vi "LSMcontroller_v59_PIzstage.vi"() -> ()   [LabVIEW 2015] (continued)
                            n1347 = call "reset AO_DO_v3.vi"() -> ()  [unwired: 12 in]
                            n1348 = property on="Start" class="Bool (strict)"("Val(Sgnl)"=w3765) -> ()  [unwired: 2 in, 2 out]
                            n1349 = property on="Start" class="Bool (strict)"("Visible"=TRUE, "DisabledEnum"=T7."Enabled" ("Disabled")) -> ()  [unwired: 2 in, 2 out]
                            n1350 = property on="Stop" class="Bool (strict)"("Val(Sgnl)"=w3765) -> ()  [unwired: 2 in, 2 out]
                            n1351 = property on="Stop" class="Bool (strict)"("Visible"=FALSE, "DisabledEnum"=T7."Disabled" ("Disabled")) -> ()  [unwired: 2 in, 2 out]
                          }
                        }
                      }
                      frame "Line" {
                      }
                      frame "Resonant Ellipse", "freeform contour" {
                        n1352 = stacked-sequence {
                          seq-local: [w3789 _ _ _ _ _ _ _ _ _ _] -> [_ _ w4634 _ _ w4647 w4714 _ _ w5074 _]
                          seq-local: [w3788 _ _ _ _ _ _ _ _ _ _] -> [_ _ _ _ _ _ _ _ w4761 _ _]
                          seq-local: [w3787 _ _ _ _ _ _ _ _ _ _] -> [_ _ _ _ _ _ _ _ w4760 _ _]
                          seq-local: [w3786 _ _ _ _ _ _ _ _ _ _] -> [_ _ _ _ _ _ _ _ w4763 _ _]
                          seq-local: [w3785 _ _ _ _ _ _ _ _ _ _] -> [_ _ _ _ _ _ _ _ w4759 _ _]
                          seq-local: [w3784 _ _ _ _ _ _ _ _ _ _] -> [_ _ _ _ _ _ _ _ w4758 _ _]
                          seq-local: [w3783 _ _ _ _ _ _ _ _ _ _] -> [_ _ _ _ _ _ _ _ w4762 _ _]
                          seq-local: [w3782 _ _ _ _ _ _ _ _ _ _] -> [_ _ _ _ _ _ _ _ w4757 _ _]
                          seq-local: [w3781 _ _ _ _ _ _ _ _ _ _] -> [_ _ _ _ _ _ _ _ w4756 _ _]
                          seq-local: [w3780 _ _ _ _ _ _ _ _ _ _] -> [_ _ _ _ _ _ _ _ w4751 _ _]
                          seq-local: [w3779 _ _ _ _ _ _ _ _ _ _] -> [_ _ _ _ _ _ _ _ w4750 _ _]
                          seq-local: [w3778 _ _ _ _ _ _ _ _ _ _] -> [_ _ _ _ _ _ _ _ w4755 _ _]
                          seq-local: [w3777 _ _ _ _ _ _ _ _ _ _] -> [_ _ _ _ _ _ _ _ w4754 _ _]
                          seq-local: [w3776 _ _ _ _ _ _ _ _ _ _] -> [_ _ _ _ _ _ _ _ w4753 _ _]
                          seq-local: [w3775 _ _ _ _ _ _ _ _ _ _] -> [_ _ _ _ _ _ _ _ w4752 _ _]
                          frame #0 {
                            n1353 = local read "save\ndata"() -> (w3790:bool)
                            n1354 = Get Date/Time In Seconds() -> (seconds since 1Jan1904=w3791:timestamp)
                            n1355 = case shown="False" w3790 {
                              tunnel: w3791 -> [w3792 w3794]
                              tunnel: [w3792 w3793] -> w3789
                              frame False {
                              }
                              frame True {
                                n1356 = call "createdatafolder.vi"("timestamp in"=w3794) -> ("current data path"=w3795:path, "timestamp out"=w3793:timestamp)
                                n1357 = local write "data dir"(w3795) -> ()
                              }
                            }
                            n1358 = stacked-sequence {
                              tunnel: w3789 -> [w3801 _ _ _ _ _ _ _ _]
                              tunnel: [_ _ _ _ _ _ w3939 _ _] -> w3788
                              tunnel: [_ _ _ _ _ _ w3938 _ _] -> w3787
                              tunnel: [_ _ _ _ _ _ w3937 _ _] -> w3786
                              tunnel: [_ _ _ _ _ _ w3936 _ _] -> w3785
                              tunnel: [_ _ _ _ _ _ w3935 _ _] -> w3784
                              tunnel: [_ _ _ _ _ _ w3934 _ _] -> w3783
                              tunnel: [_ _ _ _ _ _ w3933 _ _] -> w3782
                              tunnel: [_ _ _ _ _ _ w3932 _ _] -> w3781
                              tunnel: [_ _ _ _ _ _ w3931 _ _] -> w3780
                              tunnel: [_ _ _ _ _ _ w3930 _ _] -> w3779
                              tunnel: [_ _ _ _ _ _ w3929 _ _] -> w3778
                              tunnel: [_ _ _ _ _ _ w3928 _ _] -> w3777
                              tunnel: [_ _ _ _ _ _ w3927 _ _] -> w3776
                              tunnel: [_ _ _ _ _ _ w3926 _ _] -> w3775
                              frame #0 {
                                n1359 = local write "graphtab"(T5."timetrace" ("graphtab")) -> ()
                                n1360 = local read "AI channels"() -> (w3805:i32[])
                                n1361 = local read "CI channels"() -> (w3806:i32[])
                                n1362 = property on="Stop" class="Bool (strict)"("Visible"=TRUE, "DisabledEnum"=T7."Enabled" ("Disabled")) -> ()  [unwired: 2 in, 2 out]
                                n1363 = property on="Start" class="Bool (strict)"("Visible"=FALSE, "DisabledEnum"=T7."Disabled and Grayed Out" ("Disabled")) -> ()  [unwired: 2 in, 2 out]
                                n1364 = Format Date/Time String(time format string (%c)="%Y%m%d", seconds (now)=w3801) -> (date/time string=w3800:string)  [unwired: 1 in]
                                n1365 = Format Date/Time String(time format string (%c)="%H%M%S", seconds (now)=w3801) -> (date/time string=w3799:string)  [unwired: 1 in]
                                n1366 = call "2pparameters.vi"("command"="get") -> ("params out"=w3808:T11)  [unwired: 1 in]
                                n1367 = Bundle By Name(cluster=w3808, "aAI"=w3805, "aCI"=w3806, "type"="Timetrace", "date"=w3800, "time"=w3799) -> (w3807:T11)
                                n1368 = call "X-array-databuffer.vi"("command"=enum16{"get", "set", "clear", "append"}."clear") -> ()  [unwired: 3 in, 2 out]
                                n1369 = call "Y-array-databuffer.vi"("command"=enum16{"get", "set", "clear", "append"}."clear") -> ()  [unwired: 3 in, 2 out]
                                n1370 = call "2pparameters.vi"("Params in"=w3807, "command"="set") -> ()  [unwired: 1 out]
                                n1371 = call "CH1-1D-temp.vi"("command"=enum16{"get", "set", "clear", "append"}."clear") -> ()  [unwired: 3 in, 2 out]
                                n1372 = call "CH2-1D-temp.vi"("command"=enum16{"get", "set", "clear", "append"}."clear") -> ()  [unwired: 3 in, 2 out]
                                n1373 = call "allAI-temp.vi"("command"=enum16{"get", "set", "clear", "append"}."clear") -> ()  [unwired: 3 in, 2 out]
                              }
                              frame #1 {
                                n1374 = call "configuration.vi"("command"="get") -> ("config out"=w3825:T12)  [unwired: 2 in, 1 out]
                                n1375 = Unbundle By Name(w3825) -> ("CI names"=w3826:string[], "AI names"=w3827:string[])
                                n1376 = call "2pparameters.vi"("command"="get") -> ("params out"=w3821:T11)  [unwired: 1 in]
                                n1377 = Unbundle By Name(w3821) -> ("aCI"=w3822:i32[], "aAI"=w3823:i32[])
                                n1378 = for {
                                tunnel: w3822 -> [w3837] mode=indexing
                                tunnel: w3826 -> [w3838]
                                tunnel: [w3836] -> w3828 mode=indexing
                                n1379 = Index Array(array=w3838, index=w3837) -> (element=w3836:string)
                                }
                                n1380 = for {
                                tunnel: w3823 -> [w3834] mode=indexing
                                tunnel: w3827 -> [w3835]
                                tunnel: [w3833] -> w3829 mode=indexing
                                n1381 = Index Array(array=w3835, index=w3834) -> (element=w3833:string)
                                }
                                n1382 = Build Array (concatenate)(w3828, w3829) -> (w3819:string[])
                                n1383 = for {
                                tunnel: w3819 -> [w3831] mode=indexing
                                tunnel: [w3830] -> w3818 mode=indexing
                                i -> [w3832]
                                n1384 = Bundle("String"=w3831, w3832) -> (w3830:cluster{"String":string, i32})  [unwired: 1 in]
                                }
                                n1385 = property on="graph1list" class="Ring (strict)"("StringsAndValues[]"=w3818) -> ()  [unwired: 2 in, 2 out]
                                n1386 = property on="graph2list" class="Ring (strict)"("StringsAndValues[]"=w3818) -> ()  [unwired: 2 in, 2 out]
                              }
                              frame #2 {
                                n1387 = call "2pparameters.vi"("command"="get") -> ("params out"=w3841:T11)  [unwired: 1 in]
                                n1388 = Unbundle By Name(w3841) -> ("auto OD"=w3839:bool, "autoshutter"=w3842:bool)
                                n1389 = case shown="True" w3839 {
                                frame False {
                                }
                                frame True {
                                n1390 = call "configuration.vi"("command"="get") -> ("config out"=w3845:T12)  [unwired: 2 in, 1 out]
                                n1391 = Unbundle By Name(w3845) -> ("contour OD"=w3846:u16)
                                n1392 = local read "ODfilt"() -> (w3843:u16)
                                n1393 = call "filterwheelcontrol_nothorlabslib.vi"("Current OD filt"=w3843, "New ODfilt"=w3846) -> ()  [unwired: 1 in]
                                }
                                }
                                n1394 = case shown="True" w3842 {
                                frame False {
                                }
                                frame True {
                                n1395 = call "shuttercontrol.vi"("command"="close") -> ()  [unwired: 1 in, 1 out]
                                }
                                }
                              }
                              frame #3 {
                                n1396 = local read "Vy-min draw"() -> (w3855:dbl)
                                n1397 = local read "Vy-max draw"() -> (w3854:dbl)
                                n1398 = local read "Vx-min draw"() -> (w3857:dbl)
                                n1399 = local read "Vx-max draw"() -> (w3856:dbl)
                                n1400 = local read "xpixels ref"() -> (w3853:i32)
                                n1401 = local read "ypixels ref"() -> (w3852:i32)
                                n1402 = local read "ROI Type"() -> (w3851:u16)
                                n1403 = local read "srateAODOtt"() -> (w3874:dbl)
                                n1404 = local read "# of frames"() -> (w3879:i32)
                                n1405 = local read "refreshtime"() -> (w3871:dbl)
                                n1406 = local read "Pel"() -> (w3850:dbl)
                                n1407 = local read "bin"() -> (w3877:dbl)
                                n1408 = local read "Override AI buffer"() -> (w3848:bool)
                                n1409 = local read "finite samples"() -> (w3886:bool)
                                n1410 = local read "srateAODOtt"() -> (w3873:dbl)
                                n1411 = local read "srateAODOtt"() -> (w3880:dbl)
                                n1412 = local read "continuous"() -> (w3885:bool)
                                n1413 = local read "Angle ref"() -> (w3858:dbl)
                                n1414 = local read "wavdet"() -> (w3887:bool)
                                n1415 = local read "Vx-ref"() -> (w3882:dbl)
                                n1416 = local read "Vy-ref"() -> (w3884:dbl)
                                n1417 = local read "avpp"() -> (w3883:i32)
                                n1418 = call "tt_timeandsamples.vi"("bin"=w3877, "refreshtime"=w3871, "srateAODOtt"=w3874, "tot#ofsamples"=w3879) -> ("refreshrate"=w3875:dbl, "refreshbuffer"=w3876:i32, "timetracecycles"=w3881:i32)  [unwired: 5 in]
                                n1419 = local read "bin"() -> (w3878:dbl)
                                n1420 = call "2pparameters.vi"("command"="get") -> ("params out"=w3890:T11)  [unwired: 1 in]
                                n1421 = Bundle By Name(cluster=w3890, "Drawing Mode"=w3851, "measpoints"=w3879, "tt_cycles"=w3881, "refreshbuffer"=w3876, "refreshrate"=w3875, "Vx-ref"=w3882, "Vy-ref"=w3884, "srate"=w3873, "finite"=w3886, "cont"=w3885, "wavdet"=w3887, "avpp"=w3883, "srateAODO"=w3880, "bufferAI"=w3876, "bin"=w3878, "Angle Img"=w3858, "Vxminref"=w3857, "Vxmaxref"=w3856, "Vyminref"=w3855, "Vymaxref"=w3854, "Xpixels Img"=w3853, "Ypixels Img"=w3852, "Pel"=w3850, "Vz-reset"=0.0, "AIoverride"=w3848) -> (w3888:T11)
                                n1422 = Reciprocal(x=w3875) -> (1/x=w3872:dbl)
                                n1423 = local write "refreshtime"(w3872) -> ()
                                n1424 = call "2pparameters.vi"("Params in"=w3888, "command"="set") -> ()  [unwired: 1 out]
                                n1425 = local read "Voltage Clamp"() -> (w3865:bool)
                                n1426 = local read "Current Clamp"() -> (w3866:bool)
                                n1427 = local read "Vholding (mV)"() -> (w3860:sgl)
                                n1428 = local read "CC_ICgain"() -> (w3864:dbl)
                                n1429 = local read "OCgain"() -> (w3861:sgl)
                                n1430 = local read "holdon"() -> (w3859:bool)
                                n1431 = call "patchparameters.vi"("command"="get") -> ("Params out"=w3868:T14)  [unwired: 1 in]
                                n1432 = Bundle By Name(cluster=w3868, "VC"=w3865, "CC"=w3866, "CC_icg (pA/mv)"=w3864, "VC_icg (mV/mV)"=10.0, "OCG (mV/pA)"=w3861, "OVG (mV/mV)"=0.1, "Vhold (mV)"=w3860, "holdon"=w3859) -> (w3867:T14)
                                n1433 = call "patchparameters.vi"("Params in"=w3867, "command"="set") -> ()  [unwired: 1 out]
                              }
                              frame #4 {
                                n1434 = call "2pparameters.vi"("command"="get") -> ("params out"=w3906:T11)  [unwired: 1 in]
                                n1435 = Unbundle By Name(w3906) -> ("srateAODO"=w3907:sgl, "Angle Img"=w3908:dbl, "Angle draw"=w3909:dbl, "Vxmaxref"=w3910:dbl, "Vxminref"=w3911:dbl, "Xpixels Img"=w3912:i32, "Ypixels Img"=w3913:i32, "Vymaxref"=w3914:dbl, "Vxminref"=w3915:dbl, "Drawing Mode"=w3916:u16, "Pel"=w3917:sgl)
                                n1436 = Add(x=w3908, y=w3909) -> (x+y=w3892:dbl)
                                n1437 = call "ROI-databuffer.vi"("command"=enum16{"get", "set", "clear", "append"}."get") -> ("array out"=w3900:cluster{"x":sgl, "y":sgl}[])  [unwired: 4 in]
                                n1438 = call "ScanningWaveform_v4.vi"("Vy-min"=w3915, "Vy-max"=w3914, "yPixels/tPixels"=w3913, "xPixels/rPixels"=w3912, "Vx-min"=w3911, "Vx-max"=w3910, "Drawing Mode"=w3916, "Angle"=w3892, "AOrate"=w3907, "Points"=w3900, "points in ellipse"=w3917) -> ("numPixels"=w3893:dbl, "Y-WaveArray"=w3894:dbl[], "P"=w3899:dbl, "X-WaveArray"=w3895:dbl[])  [unwired: 5 in]
                                n1439 = call "Y-array-databuffer.vi"("array in"=w3894, "command"=enum16{"get", "set", "clear", "append"}."set") -> ()  [unwired: 2 in, 2 out]
                                n1440 = call "X-array-databuffer.vi"("array in"=w3895, "command"=enum16{"get", "set", "clear", "append"}."set") -> ()  [unwired: 2 in, 2 out]
                                n1441 = call "2pparameters.vi"("command"="get") -> ("params out"=w3904:T11)  [unwired: 1 in]
                                n1442 = Bundle By Name(cluster=w3904, "P"=w3899, "sAOxy"=w3893, "Pel"=w3893) -> (w3896:T11)
                                n1443 = call "2pparameters.vi"("Params in"=w3896, "command"="set") -> ()  [unwired: 1 out]
                              }
                              frame #5 {
                                n1444 = call "X-array-databuffer.vi"("command"=enum16{"get", "set", "clear", "append"}."get") -> ("array out"=w3920:dbl[])  [unwired: 3 in, 1 out]
                                n1445 = call "Y-array-databuffer.vi"("command"=enum16{"get", "set", "clear", "append"}."get") -> ("array out"=w3923:dbl[])  [unwired: 3 in, 1 out]
                                n1446 = Index Array(array=w3920, index=0) -> (element=w3919:dbl)
                                n1447 = Index Array(array=w3923, index=0) -> (element=w3918:dbl)
                                n1448 = call "setposition.vi"("Vy"=w3918, "Vx"=w3919) -> ()  [unwired: 1 in]
                              }
                              frame #6 {
                                # "rem2Ps"
                                # "A2Ps"
                                # "Al"
                                # "Rl"
                                n1449 = stacked-sequence {
                                seq-local: [w3944 _ _ _ _ _ _ _ _ _ _] -> [_ w4056 _ w4117 _ w4203 _ _ _ _ _]
                                seq-local: [w3945 _ _ _ _ _ _ _ _ _ _] -> [_ w4057 w4067 _ w4172 _ _ _ _ _ _]
                                seq-local: [_ _ w4066 _ _ _ _ _ _ _ _] -> [_ _ _ _ w4166 _ _ _ _ _ _]
                                seq-local: [_ _ _ w4116 _ _ _ _ _ _ _] -> [_ _ _ _ _ w4202 _ _ _ _ _]
                                seq-local: [w3941 _ _ _ _ _ _ _ _ _ _] -> [_ w4053 _ _ _ _ _ _ w4388 w4456 _]
                                seq-local: [w3940 _ _ _ _ _ _ _ _ _ _] -> [_ w4052 _ _ _ _ _ _ w4389 w4457 _]
                                seq-local: [w3947 _ _ _ _ _ _ _ _ _ _] -> [_ _ _ _ _ _ w4241 _ w4387 w4455 _]
                                seq-local: [w3943 _ _ _ _ _ _ _ _ _ _] -> [_ w4051 _ _ _ _ w4240 w4308 _ _ _]
                                seq-local: [w3942 _ _ _ _ _ _ _ _ _ _] -> [_ w4050 _ _ _ _ w4239 w4307 _ _ _]
                                seq-local: [w3946 _ _ _ _ _ _ _ _ _ _] -> [_ _ _ _ _ _ w4238 w4306 _ _ _]
                                tunnel: [_ _ w4065 _ _ _ _ _ _ _ _] -> w3938
                                tunnel: [_ _ w4064 _ _ _ _ _ _ _ _] -> w3939
                                tunnel: [w3945 _ _ _ _ _ _ _ _ _ _] -> w3937
                                tunnel: [w3944 _ _ _ _ _ _ _ _ _ _] -> w3934
                                tunnel: [_ _ _ w4115 _ _ _ _ _ _ _] -> w3935
                                tunnel: [_ _ _ w4114 _ _ _ _ _ _ _] -> w3936
                                tunnel: [w3943 _ _ _ _ _ _ _ _ _ _] -> w3929
                                tunnel: [w3942 _ _ _ _ _ _ _ _ _ _] -> w3928
                                tunnel: [_ _ _ _ _ _ w4237 _ _ _ _] -> w3927
                                tunnel: [_ _ _ _ _ _ _ w4305 _ _ _] -> w3926
                                tunnel: [w3941 _ _ _ _ _ _ _ _ _ _] -> w3930
                                tunnel: [w3940 _ _ _ _ _ _ _ _ _ _] -> w3931
                                tunnel: [_ _ _ _ _ _ _ _ w4386 _ _] -> w3932
                                tunnel: [_ _ _ _ _ _ _ _ _ w4454 _] -> w3933
                                frame #0 {
                                # "for a next version, give ome thought to\nthe possibilit of intermittently updating the\nwaveforms. it will have to be a calculation\nbased on speed of CPU and program on the one hand\nand length of measurement on the other. but then it should be possible, in principle, to \nupdate the waveform on the fly and that way cut up a longer measurement in smaller parts."
                                n1450 = stacked-sequence {
                                tunnel: [w3948 _ _ _] -> w3945
                                tunnel: [_ w3960 _ _] -> w3944
                                tunnel: [_ _ _ w4017] -> w3940
                                tunnel: [_ _ _ w4016] -> w3941
                                tunnel: [_ _ _ w4015] -> w3947
                                tunnel: [_ _ w3975 _] -> w3943
                                tunnel: [_ _ w3974 _] -> w3942
                                tunnel: [_ _ w3973 _] -> w3946
                                frame #0 {
                                n1451 = call "configuration.vi"("command"="get") -> ("config out"=w3950:T12)  [unwired: 2 in, 1 out]
                                n1452 = Unbundle By Name(w3950) -> ("Voltage to Xgalvo"=w3949:i32)
                                n1453 = call "2pparameters.vi"("command"="get") -> ("params out"=w3954:T11)  [unwired: 1 in]
                                n1454 = in-place {
                                in-place-border: w3949 -> [w3959]
                                in-place-border: [w3956] -> w3948
                                n1455 = in-place-cluster #23(w3954) -> ("aAO"=w3958:u32[])
                                n1456 = call "add channel to active arrayv2.vi"("line array in"=w3958, "line to add"=w3959) -> ("line array out"=w3957:u32[], "addition"=w3956:bool)  [unwired: 1 out]
                                n1457 = in-place-cluster #23("aAO"=w3957) -> (w3952:T11)
                                }
                                n1458 = call "2pparameters.vi"("Params in"=w3952, "command"="set") -> ()  [unwired: 1 out]
                                }
                                frame #1 {
                                n1459 = call "configuration.vi"("command"="get") -> ("config out"=w3962:T12)  [unwired: 2 in, 1 out]
                                n1460 = Unbundle By Name(w3962) -> ("Voltage to Ygalvo"=w3961:i32)
                                n1461 = call "2pparameters.vi"("command"="get") -> ("params out"=w3966:T11)  [unwired: 1 in]
                                n1462 = in-place {
                                in-place-border: w3961 -> [w3971]
                                in-place-border: [w3968] -> w3960
                                n1463 = in-place-cluster #24(w3966) -> ("aAO"=w3970:u32[])
                                n1464 = call "add channel to active arrayv2.vi"("line array in"=w3970, "line to add"=w3971) -> ("line array out"=w3969:u32[], "addition"=w3968:bool)  [unwired: 1 out]
                                n1465 = in-place-cluster #24("aAO"=w3969) -> (w3964:T11)
                                }
                                n1466 = call "2pparameters.vi"("Params in"=w3964, "command"="set") -> ()  [unwired: 1 out]
                                }
                                frame #2 {
                                n1467 = call "2pparameters.vi"("command"="get") -> ("params out"=w3977:T11)  [unwired: 1 in]
                                n1468 = Unbundle By Name(w3977) -> ("autoshutter"=w3976:bool, "wavdet"=w3972:bool)
                                n1469 = case shown="False" w3976 {
                                tunnel: [w3982 w4002] -> w3975
                                tunnel: [w3981 FALSE ("removal")] -> w3974
                                tunnel: [w3980 w4000] -> w3973
                                tunnel: w3972 -> [w3979 _]
                                frame False {
                                n1470 = case shown="False" w3979 {
                                tunnel: [FALSE ("addition") FALSE ("addition")] -> w3982
                                tunnel: [w3984 FALSE ("removal")] -> w3981
                                tunnel: [w3983 _] -> w3980
                                frame False {
                                n1471 = call "configuration.vi"("command"="get") -> ("config out"=w3990:T12)  [unwired: 2 in, 1 out]
                                n1472 = Unbundle By Name(w3990) -> ("2P shutter"=w3987:i32)
                                n1473 = call "2pparameters.vi"("command"="get") -> ("params out"=w3988:T11)  [unwired: 1 in]
                                n1474 = in-place {
                                in-place-border: w3987 -> [w3997]
                                in-place-border: [w3994] -> w3984
                                in-place-border: [w3993] -> w3983
                                n1475 = in-place-cluster #25(w3988) -> ("aDO"=w3996:u32[])
                                n1476 = call "remove channel from active arrayv2.vi"("line array in"=w3996, "line to remove"=w3997) -> ("line array out"=w3995:u32[], "removal"=w3994:bool, "index"=w3993:i32)
                                n1477 = in-place-cluster #25("aDO"=w3995) -> (w3985:T11)
                                }
                                n1478 = call "2pparameters.vi"("Params in"=w3985, "command"="set") -> ()  [unwired: 1 out]
                                }
                                frame True {
                                }
                                }
                                }
                                frame True {
                                n1479 = call "configuration.vi"("command"="get") -> ("config out"=w4004:T12)  [unwired: 2 in, 1 out]
                                n1480 = call "2pparameters.vi"("command"="get") -> ("params out"=w4008:T11)  [unwired: 1 in]
                                n1481 = Unbundle By Name(w4004) -> ("2P shutter"=w4003:i32)
                                n1482 = in-place {
                                in-place-border: w4003 -> [w4014]
                                in-place-border: [w4011] -> w4002
                                in-place-border: [w4010] -> w4000
                                n1483 = in-place-cluster #26(w4008) -> ("aDO"=w4013:u32[])
                                n1484 = call "add channel to active arrayv2.vi"("line array in"=w4013, "line to add"=w4014) -> ("line array out"=w4012:u32[], "addition"=w4011:bool, "index"=w4010:i32)
                                n1485 = in-place-cluster #26("aDO"=w4012) -> (w4006:T11)
                                }
                                n1486 = call "2pparameters.vi"("Params in"=w4006, "command"="set") -> ()  [unwired: 1 out]
                                }
                                }
                                }
                                frame #3 {
                                n1487 = local read "Measurement"() -> (w4018:T4)
                                n1488 = To Unsigned Long Integer(number=w4018) -> (unsigned 32bit integer=w4019:u32)
                                n1489 = case shown="5..7" w4019 {
                                tunnel: [FALSE ("addition") w4037] -> w4017
                                tunnel: [w4022 FALSE ("removal")] -> w4016
                                tunnel: [w4020 w4035] -> w4015
                                frame 0..4, Default {
                                n1490 = call "configuration.vi"("command"="get") -> ("config out"=w4028:T12)  [unwired: 2 in, 1 out]
                                n1491 = Unbundle By Name(w4028) -> ("LT timestamp"=w4025:u32)
                                n1492 = call "2pparameters.vi"("command"="get") -> ("params out"=w4026:T11)  [unwired: 1 in]
                                n1493 = in-place {
                                in-place-border: w4025 -> [w4034]
                                in-place-border: [w4031] -> w4022
                                in-place-border: [w4030] -> w4020
                                n1494 = in-place-cluster #27(w4026) -> ("aDO"=w4033:u32[])
                                n1495 = call "remove channel from active arrayv2.vi"("line array in"=w4033, "line to remove"=w4034) -> ("line array out"=w4032:u32[], "removal"=w4031:bool, "index"=w4030:i32)
                                n1496 = in-place-cluster #27("aDO"=w4032) -> (w4023:T11)
                                }
                                n1497 = call "2pparameters.vi"("Params in"=w4023, "command"="set") -> ()  [unwired: 1 out]
                                }
                                frame 5..7 {
                                n1498 = call "configuration.vi"("command"="get") -> ("config out"=w4043:T12)  [unwired: 2 in, 1 out]
                                n1499 = Unbundle By Name(w4043) -> ("LT timestamp"=w4040:u32)
                                n1500 = call "2pparameters.vi"("command"="get") -> ("params out"=w4041:T11)  [unwired: 1 in]
                                n1501 = in-place {
                                in-place-border: w4040 -> [w4049]
                                in-place-border: [w4046] -> w4037
                                in-place-border: [w4045] -> w4035
                                n1502 = in-place-cluster #28(w4041) -> ("aDO"=w4048:u32[])
                                n1503 = call "add channel to active arrayv2.vi"("line array in"=w4048, "line to add"=w4049) -> ("line array out"=w4047:u32[], "addition"=w4046:bool, "index"=w4045:i32)
                                n1504 = in-place-cluster #28("aDO"=w4047) -> (w4038:T11)
                                }
                                n1505 = call "2pparameters.vi"("Params in"=w4038, "command"="set") -> ()  [unwired: 1 out]
                                }
                                }
                                }
                                }
                                }
                                frame #1 {
                                n1506 = Or(x=w4056, y=w4057) -> (x .or. y?=w4055:bool)
                                n1507 = case shown="True" w4055 {
                                frame False {
                                }
                                frame True {
                                # "update GUI"
                                n1508 = call "Used AO lines.vi"() -> ("used AO names"=w4061:string[], "used AO lines"=w4063:tag[])  [unwired: 2 in]
                                n1509 = control-ref of="Analog Lines Plot"() -> (w4062:refnum<vi>)
                                n1510 = local write "Analog Used Lines"(w4063) -> ()
                                n1511 = local write "Analog Used Names"(w4061) -> ()
                                n1512 = call "prepAOWaveplot.vi"("WaveformGraph in"=w4062, "Analog Used Names"=w4061) -> ()  [unwired: 1 in]
                                }
                                }
                                n1513 = Compound Arithmetic op=OR(w4053, w4052, w4051, w4050) -> (w4054:bool)
                                n1514 = case shown="True" w4054 {
                                frame False {
                                }
                                frame True {
                                n1515 = control-ref of="Digital Lines Plot"() -> (w4058:refnum<vi>)
                                n1516 = call "Used DO lines.vi"() -> ("used DO names"=w4059:string[], "used DO lines"=w4060:tag[])  [unwired: 2 in]
                                n1517 = local write "Digital Used Lines"(w4060) -> ()
                                n1518 = local write "Digital Used Names"(w4059) -> ()
                                n1519 = call "prepDOWaveplot.vi"("DigitalGraph in"=w4058, "used DO names"=w4059) -> ()  [unwired: 1 in]
                                }
                                }
                                }
                                frame #2 {
                                n1520 = case shown="False" w4067 {
                                tunnel: [w4070 w4096] -> w4066
                                tunnel: [w4069 w4094] -> w4065
                                tunnel: [w4068 _] -> w4064
                                frame False {
                                n1521 = stacked-sequence {
                                seq-local: [w4072 _] -> [_ w4087]
                                tunnel: [w4072 _] -> w4070
                                tunnel: [w4075 _] -> w4069
                                tunnel: [w4071 _] -> w4068
                                frame #0 {
                                n1522 = call "configuration.vi"("command"="get") -> ("config out"=w4083:T12)  [unwired: 2 in, 1 out]
                                n1523 = call "waveformparamsv2.vi"("command"="get") -> ("Params out"=w4077:T15)  [unwired: 4 in, 2 out]
                                n1524 = Unbundle By Name(w4083) -> ("Voltage to Xgalvo"=w4084:i32)
                                n1525 = call "2pparameters.vi"("command"="get") -> ("params out"=w4080:T11)  [unwired: 1 in]
                                n1526 = Unbundle By Name(w4077) -> ("AO parameters"=w4076:T16)
                                n1527 = Unbundle By Name(w4080) -> ("aAO"=w4081:u32[])
                                n1528 = call "waveformsAObuffer.vi"("command"="get") -> ("AO wf out"=w4073:waveform(dbl)[])  [unwired: 1 in]
                                n1529 = Search 1D Array(1D array=w4081, element=w4084) -> (index of element=w4072:i32)  [unwired: 1 in]
                                n1530 = Index Array(array=w4073, index=w4072) -> (element=w4071:waveform(dbl))
                                n1531 = Index Array(array=w4076, index=w4072) -> (element=w4075:T17)
                                }
                                frame #1 {
                                w4088 = 0.0 ("Step size (V)")
                                n1532 = local read "Meastab"() -> (w4086:enum32{"X-Y Image", "Linescan", "Timetrace"})
                                n1533 = case shown="\"X-Y Image\", Default" w4086 {
                                tunnel: [w4090 w4091] -> w4085
                                frame "X-Y Image", Default {
                                n1534 = local read "Sampling rate"() -> (w4090:dbl)
                                }
                                frame "Timetrace" {
                                n1535 = local read "srateAODOtt"() -> (w4091:dbl)
                                }
                                }
                                n1536 = call "replace AO XYwfparam.vi"("Baseline (V)"=w4088, "Start amplitude (V)"=w4088, "Cycles"=w4088, "Repeats"=w4088, "index of AO wave"=w4087, "Step size (V)"=w4088, "DC (%)"=w4088, "Sampling frequency (Hz)"=w4085, "Period (ms)"=w4088, "Cycle length (s)"=w4088, "Pulses"=w4088, "padding value"=w4088, "Matlab wave name"=path "xwave") -> ()  [unwired: 3 in]
                                }
                                }
                                }
                                frame True {
                                w4095 = 0.0 ("Repeats")
                                n1537 = local read "Meastab"() -> (w4093:enum32{"X-Y Image", "Linescan", "Timetrace"})
                                n1538 = case shown="\"X-Y Image\", Default" w4093 {
                                tunnel: [w4112 w4113] -> w4092
                                frame "X-Y Image", Default {
                                n1539 = local read "Sampling rate"() -> (w4112:dbl)
                                }
                                frame "Timetrace" {
                                n1540 = local read "srateAODOtt"() -> (w4113:dbl)
                                }
                                }
                                n1541 = call "2pparameters.vi"("command"="get") -> ("params out"=w4098:T11)  [unwired: 1 in]
                                n1542 = call "configuration.vi"("command"="get") -> ("config out"=w4101:T12)  [unwired: 2 in, 1 out]
                                n1543 = call "waveformparamsv2.vi"("command"="get") -> ("Params out"=w4109:T15)  [unwired: 4 in, 2 out]
                                n1544 = Unbundle By Name(w4101) -> ("Voltage to Xgalvo"=w4102:i32)
                                n1545 = Unbundle By Name(w4109) -> ("AO parameters"=w4106:T16)
                                n1546 = Unbundle By Name(w4098) -> ("aAO"=w4099:u32[])
                                n1547 = Search 1D Array(1D array=w4099, element=w4102) -> (index of element=w4096:i32)  [unwired: 1 in]
                                n1548 = Index Array(array=w4106, index=0) -> (element=w4107:T17)
                                n1549 = Bundle By Name(cluster=w4107, "AOtab"=-1.0 ("Repeats"), "Repeats"=w4095, "Cycles"=w4095, "Start amplitude (V)"=w4095, "Baseline (V)"=w4095, "Step size (V)"=w4095, "DC (%)"=w4095, "Sampling frequency (Hz)"=w4092, "Period (ms)"=w4095, "Offset (V)"=w4095, "Amplitude (V)"=w4095, "Frequency"=w4095, "Tri Repeats"=w4095, "phase shift (ms)"=w4095, "Pulses"=w4095, "Matlab wave file"=path "xwave", "padding value"=w4095) -> (w4094:T17)
                                n1550 = Build Array(w4094) -> (w4104:T16)
                                n1551 = call "waveformparamsv2.vi"("command"="add AO", "add AO"=w4104) -> ()  [unwired: 3 in, 3 out]
                                }
                                }
                                }
                                frame #3 {
                                n1552 = case shown="True" w4117 {
                                tunnel: [w4120 w4146] -> w4116
                                tunnel: [w4119 w4144] -> w4115
                                tunnel: [w4118 _] -> w4114
                                frame False {
                                n1553 = stacked-sequence {
                                seq-local: [w4122 _] -> [_ w4137]
                                tunnel: [w4122 _] -> w4120
                                tunnel: [w4125 _] -> w4119
                                tunnel: [w4121 _] -> w4118
                                frame #0 {
                                n1554 = call "configuration.vi"("command"="get") -> ("config out"=w4133:T12)  [unwired: 2 in, 1 out]
                                n1555 = call "waveformparamsv2.vi"("command"="get") -> ("Params out"=w4127:T15)  [unwired: 4 in, 2 out]
                                n1556 = Unbundle By Name(w4133) -> ("Voltage to Ygalvo"=w4134:i32)
                                n1557 = call "2pparameters.vi"("command"="get") -> ("params out"=w4130:T11)  [unwired: 1 in]
                                n1558 = Unbundle By Name(w4127) -> ("AO parameters"=w4126:T16)
                                n1559 = Unbundle By Name(w4130) -> ("aAO"=w4131:u32[])
                                n1560 = call "waveformsAObuffer.vi"("command"="get") -> ("AO wf out"=w4123:waveform(dbl)[])  [unwired: 1 in]
                                n1561 = Search 1D Array(1D array=w4131, element=w4134) -> (index of element=w4122:i32)  [unwired: 1 in]
                                n1562 = Index Array(array=w4123, index=w4122) -> (element=w4121:waveform(dbl))
                                n1563 = Index Array(array=w4126, index=w4122) -> (element=w4125:T17)
                                }
                                frame #1 {
                                w4138 = 0.0 ("Step size (V)")
                                n1564 = local read "Meastab"() -> (w4136:enum32{"X-Y Image", "Linescan", "Timetrace"})
                                n1565 = case shown="\"X-Y Image\", Default" w4136 {
                                tunnel: [w4140 w4141] -> w4135
                                frame "X-Y Image", Default {
                                n1566 = local read "Sampling rate"() -> (w4140:dbl)
                                }
                                frame "Timetrace" {
                                n1567 = local read "srateAODOtt"() -> (w4141:dbl)
                                }
                                }
                                n1568 = call "replace AO XYwfparam.vi"("Baseline (V)"=w4138, "Start amplitude (V)"=w4138, "Cycles"=w4138, "Repeats"=w4138, "index of AO wave"=w4137, "Step size (V)"=w4138, "DC (%)"=w4138, "Sampling frequency (Hz)"=w4135, "Period (ms)"=w4138, "Cycle length (s)"=w4138, "Pulses"=w4138, "padding value"=w4138, "Matlab wave name"=path "ywave") -> ()  [unwired: 3 in]
                                }
                                }
                                }
                                frame True {
                                w4145 = 0.0 ("Repeats")
                                n1569 = local read "Meastab"() -> (w4143:enum32{"X-Y Image", "Linescan", "Timetrace"})
                                n1570 = case shown="\"X-Y Image\", Default" w4143 {
                                tunnel: [w4162 w4163] -> w4142
                                frame "X-Y Image", Default {
                                n1571 = local read "Sampling rate"() -> (w4162:dbl)
                                }
                                frame "Timetrace" {
                                n1572 = local read "srateAODOtt"() -> (w4163:dbl)
                                }
                                }
                                n1573 = call "2pparameters.vi"("command"="get") -> ("params out"=w4148:T11)  [unwired: 1 in]
                                n1574 = call "configuration.vi"("command"="get") -> ("config out"=w4151:T12)  [unwired: 2 in, 1 out]
                                n1575 = call "waveformparamsv2.vi"("command"="get") -> ("Params out"=w4160:T15)  [unwired: 4 in, 2 out]
                                n1576 = Unbundle By Name(w4151) -> ("Voltage to Ygalvo"=w4152:i32)
                                n1577 = Unbundle By Name(w4160) -> ("AO parameters"=w4157:T16)
                                n1578 = Unbundle By Name(w4148) -> ("aAO"=w4149:u32[])
                                n1579 = Search 1D Array(1D array=w4149, element=w4152) -> (index of element=w4146:i32)  [unwired: 1 in]
                                n1580 = Index Array(array=w4157, index=0) -> (element=w4158:T17)
                                n1581 = Bundle By Name(cluster=w4158, "AOtab"=-1.0 ("Repeats"), "Repeats"=w4145, "Cycles"=w4145, "Start amplitude (V)"=w4145, "Baseline (V)"=w4145, "Step size (V)"=w4145, "DC (%)"=w4145, "Sampling frequency (Hz)"=w4142, "Period (ms)"=w4145, "Offset (V)"=w4145, "Amplitude (V)"=w4145, "Frequency"=w4145, "Tri Repeats"=w4145, "phase shift (ms)"=w4145, "Pulses"=w4145, "Matlab wave file"=path "ywave", "padding value"=w4145) -> (w4144:T17)
                                n1582 = Build Array(w4144) -> (w4155:T16)
                                n1583 = call "waveformparamsv2.vi"("command"="add AO", "add AO"=w4155) -> ()  [unwired: 3 in, 3 out]
                                }
                                }
                                }
                                frame #4 {
                                n1584 = call "2pparameters.vi"("command"="get") -> ("params out"=w4169:T11)  [unwired: 1 in]
                                n1585 = Unbundle By Name(w4169) -> ("wavdet"=w4168:bool, "Pel"=w4165:sgl, "refwfsize"=w4164:dbl, "srateAODO"=w4167:sgl)
                                n1586 = case shown="True" w4168 {
                                tunnel: [w4173 w4183] -> w4171
                                tunnel: w4167 -> [w4174 w4185]
                                tunnel: w4165 -> [_ w4181]
                                tunnel: w4164 -> [_ w4180]
                                frame False {
                                n1587 = call "X-array-databuffer.vi"("command"=enum16{"get", "set", "clear", "append"}."get") -> ("array out"=w4177:dbl[])  [unwired: 3 in, 1 out]
                                n1588 = Reciprocal(x=w4174) -> (1/x=w4175:sgl)
                                n1589 = Bundle By Name("Y"=w4177, "dt"=w4175) -> (w4173:waveform(dbl))  [unwired: 1 in]
                                }
                                frame True {
                                n1590 = To Double Precision Float(number=w4181) -> (double precision float=w4182:dbl)
                                n1591 = Divide(x=w4180, y=w4182) -> (x/y=w4179:dbl)
                                n1592 = Round Toward +Infinity(x=w4179) -> (ceil(x): smallest int >= x=w4178:dbl)
                                n1593 = call "X-array-databuffer.vi"("command"=enum16{"get", "set", "clear", "append"}."get") -> ("array out"=w4187:dbl[])  [unwired: 3 in, 1 out]
                                n1594 = Reciprocal(x=w4185) -> (1/x=w4186:sgl)
                                n1595 = for {
                                N: w4178 -> [_]
                                tunnel: w4187 -> [w4189]
                                tunnel: [w4189] -> w4184 mode=concatenating
                                }
                                n1596 = Bundle By Name("Y"=w4184, "dt"=w4186) -> (w4183:waveform(dbl))  [unwired: 1 in]
                                }
                                }
                                n1597 = case shown="True" w4172 {
                                tunnel: w4171 -> [w4191 w4197]
                                tunnel: w4166 -> [w4192 _]
                                frame False {
                                n1598 = call "waveformsAObuffer.vi"("command"="get") -> ("AO wf out"=w4195:waveform(dbl)[])  [unwired: 1 in]
                                n1599 = property on="refwf" class="Ring (strict)" props=["RingText", "Text"]() -> ()  [unwired: 2 in, 3 out]
                                n1600 = Replace Array Subset(array=w4195, new element=w4191, index=w4192) -> (w4190:waveform(dbl)[])
                                n1601 = call "waveformsAObuffer.vi"("AO wf in"=w4190, "command"="set") -> ()  [unwired: 1 out]
                                }
                                frame True {
                                n1602 = call "waveformsAObuffer.vi"("command"="get") -> ("AO wf out"=w4199:waveform(dbl)[])  [unwired: 1 in]
                                n1603 = Build Array (concatenate)(w4199, w4197) -> (w4196:waveform(dbl)[])
                                n1604 = call "waveformsAObuffer.vi"("AO wf in"=w4196, "command"="set") -> ()  [unwired: 1 out]
                                }
                                }
                                }
                                frame #5 {
                                n1605 = call "2pparameters.vi"("command"="get") -> ("params out"=w4211:T11)  [unwired: 1 in]
                                n1606 = Unbundle By Name(w4211) -> ("wavdet"=w4210:bool, "Pel"=w4208:sgl, "refwfsize"=w4209:dbl, "srateAODO"=w4204:sgl)
                                n1607 = To Double Precision Float(number=w4208) -> (double precision float=w4207:dbl)
                                n1608 = Divide(x=w4209, y=w4207) -> (x/y=w4206:dbl)
                                n1609 = Round Toward +Infinity(x=w4206) -> (ceil(x): smallest int >= x=w4205:dbl)
                                n1610 = case shown="True" w4210 {
                                tunnel: [w4215 w4221] -> w4201
                                tunnel: w4205 -> [_ w4218]
                                tunnel: w4204 -> [w4216 w4223]
                                frame False {
                                n1611 = call "Y-array-databuffer.vi"("command"=enum16{"get", "set", "clear", "append"}."get") -> ("array out"=w4213:dbl[])  [unwired: 3 in, 1 out]
                                n1612 = Reciprocal(x=w4216) -> (1/x=w4217:sgl)
                                n1613 = Bundle By Name("Y"=w4213, "dt"=w4217) -> (w4215:waveform(dbl))  [unwired: 1 in]
                                }
                                frame True {
                                n1614 = call "Y-array-databuffer.vi"("command"=enum16{"get", "set", "clear", "append"}."get") -> ("array out"=w4219:dbl[])  [unwired: 3 in, 1 out]
                                n1615 = Reciprocal(x=w4223) -> (1/x=w4224:sgl)
                                n1616 = for {
                                N: w4218 -> [_]
                                tunnel: w4219 -> [w4225]
                                tunnel: [w4225] -> w4222 mode=concatenating
                                }
                                n1617 = Bundle By Name("Y"=w4222, "dt"=w4224) -> (w4221:waveform(dbl))  [unwired: 1 in]
                                }
                                }
                                n1618 = case shown="False" w4203 {
                                tunnel: w4201 -> [w4228 w4233]
                                tunnel: w4202 -> [w4229 _]
                                frame False {
                                n1619 = call "waveformsAObuffer.vi"("command"="get") -> ("AO wf out"=w4231:waveform(dbl)[])  [unwired: 1 in]
                                n1620 = Replace Array Subset(array=w4231, new element=w4228, index=w4229) -> (w4226:waveform(dbl)[])
                                n1621 = call "waveformsAObuffer.vi"("AO wf in"=w4226, "command"="set") -> ()  [unwired: 1 out]
                                }
                                frame True {
                                n1622 = call "waveformsAObuffer.vi"("command"="get") -> ("AO wf out"=w4235:waveform(dbl)[])  [unwired: 1 in]
                                n1623 = Build Array (concatenate)(w4235, w4233) -> (w4232:waveform(dbl)[])
                                n1624 = call "waveformsAObuffer.vi"("AO wf in"=w4232, "command"="set") -> ()  [unwired: 1 out]
                                }
                                }
                                }
                                frame #6 {
                                n1625 = Build Array(w4240, w4239) -> (w4243:bool[])
                                n1626 = Boolean Array To Number(Boolean array=w4243) -> (number=w4242:u32)
                                n1627 = case shown="1" w4242 {
                                tunnel: w4241 -> [_ _ _ _]
                                tunnel: w4238 -> [_ w4266 _ w4279]
                                tunnel: [_ w4265 _ w4276] -> w4237
                                frame 1 {
                                w4253 = 0.0 ("DOtab")
                                n1628 = call "2pparameters.vi"("command"="get") -> ("params out"=w4250:T11)  [unwired: 1 in]
                                n1629 = call "waveformparamsv2.vi"("command"="get") -> ("Params out"=w4261:T15)  [unwired: 4 in, 2 out]
                                n1630 = Unbundle By Name(w4261) -> ("DO parameters"=w4259:T18)
                                n1631 = Unbundle By Name(w4250) -> ("srate"=w4246:sgl, "Pel"=w4249:sgl)
                                n1632 = To Double Precision Float(number=w4246) -> (double precision float=w4244:dbl)
                                n1633 = To Double Precision Float(number=w4246) -> (double precision float=w4245:dbl)
                                n1634 = To Double Precision Float(number=w4249) -> (double precision float=w4248:dbl)
                                n1635 = Divide(x=w4245, y=w4248) -> (x/y=w4247:dbl)
                                n1636 = Index Array(array=w4259, index=0) -> (element=w4258:T19)
                                n1637 = Bundle By Name(cluster=w4258, "Digital DC (%)"=100.0, "Digital phase"=w4253, "Digital Freq (Hz)"=w4247, "Sampling frequency (Hz)"=w4244, "Digital time offset (s)"=w4253, "padding value"=0.0, "matlab wave file"=path "2Pshutter", "DOtab"=0.0) -> (w4256:T19)
                                n1638 = Build Array(w4256) -> (w4255:T18)
                                n1639 = call "waveformparamsv2.vi"("command"="add DO", "add DO"=w4255) -> ()  [unwired: 3 in, 3 out]
                                }
                                frame 2 {
                                n1640 = call "waveformparamsv2.vi"("command"="get") -> ("Params out"=w4268:T15)  [unwired: 4 in, 2 out]
                                n1641 = in-place {
                                in-place-border: w4266 -> [w4272]
                                in-place-border: [w4271] -> w4265
                                n1642 = in-place-cluster #29(w4268) -> ("DO parameters"=w4274:T18)
                                n1643 = Delete From Array(array=w4274, length=1, index=w4272) -> (deleted portion=w4271:T18, array with subset deleted=w4273:T18)
                                n1644 = in-place-cluster #29("DO parameters"=w4273) -> (w4267:T15)
                                }
                                n1645 = call "waveformparamsv2.vi"("command"="set", "Params in"=w4267) -> ()  [unwired: 3 in, 3 out]
                                }
                                frame 3, Default {
                                }
                                frame 0 {
                                n1646 = call "2pparameters.vi"("command"="get") -> ("params out"=w4281:T11)  [unwired: 1 in]
                                n1647 = Unbundle By Name(w4281) -> ("wavdet"=w4278:bool, "autoshutter"=w4280:bool)
                                n1648 = case shown="True" w4280 {
                                tunnel: w4279 -> [_ w4285]
                                tunnel: w4278 -> [_ w4284]
                                tunnel: [_ w4283] -> w4277
                                frame False {
                                }
                                frame True {
                                n1649 = case shown="False" w4284 {
                                tunnel: w4285 -> [w4287 _]
                                tunnel: [w4286 _] -> w4283
                                frame False {
                                n1650 = stacked-sequence {
                                tunnel: w4287 -> [w4289 w4303]
                                tunnel: [w4288 _] -> w4286
                                frame #0 {
                                n1651 = call "waveformparamsv2.vi"("command"="get") -> ("Params out"=w4291:T15)  [unwired: 4 in, 2 out]
                                n1652 = Unbundle By Name(w4291) -> ("DO parameters"=w4290:T18)
                                n1653 = Index Array(array=w4290, index=w4289) -> (element=w4288:T19)
                                }
                                frame #1 {
                                w4302 = 0.0 ("padding value")
                                n1654 = call "2pparameters.vi"("command"="get") -> ("params out"=w4300:T11)  [unwired: 1 in]
                                n1655 = Unbundle By Name(w4300) -> ("srate"=w4297:sgl, "Pel"=w4299:sgl)
                                n1656 = To Double Precision Float(number=w4297) -> (double precision float=w4295:dbl)
                                n1657 = To Double Precision Float(number=w4297) -> (double precision float=w4296:dbl)
                                n1658 = To Double Precision Float(number=w4299) -> (double precision float=w4298:dbl)
                                n1659 = Divide(x=w4296, y=w4298) -> (x/y=w4294:dbl)
                                n1660 = call "replace DO wf param.vi"("Digital Freq (Hz)"=w4294, "Digital DC (%)"=100.0, "Digital phase"=w4302, "Sampling frequency (Hz)"=w4295, "Digital time offset (s)"=w4302, "index of DO wave"=w4303, "padding value"=w4302, "matlab wave file"=path "2Pshutter" ("matlab wave number")) -> ()  [unwired: 3 in]
                                }
                                }
                                }
                                frame True {
                                }
                                }
                                }
                                }
                                n1661 = Build Array(w4277) -> (w4276:T18)
                                }
                                }
                                }
                                frame #7 {
                                n1662 = Build Array(w4308, w4307) -> (w4310:bool[])
                                n1663 = Boolean Array To Number(Boolean array=w4310) -> (number=w4309:u32)
                                n1664 = case shown="0" w4309 {
                                tunnel: w4306 -> [_ w4352 _ w4359]
                                tunnel: [_ w4351 _ w4357] -> w4305
                                frame 1 {
                                n1665 = call "2pparameters.vi"("command"="get") -> ("params out"=w4317:T11)  [unwired: 1 in]
                                n1666 = Unbundle By Name(w4317) -> ("wavdet"=w4318:bool, "Pel"=w4320:sgl, "refwfsize"=w4321:dbl, "srateAODO"=w4319:sgl)
                                n1667 = call "waveformsDObuffer.vi"("command"="get") -> ("DO wf out"=w4313:digitalwaveform[])  [unwired: 1 in]
                                n1668 = case shown="False" w4318 {
                                tunnel: [w4326 w4336] -> w4315
                                tunnel: w4319 -> [w4331 w4347]
                                tunnel: w4320 -> [w4325 w4340]
                                tunnel: w4321 -> [_ w4344]
                                frame False {
                                w4329 = u16 0 items=["unsigned binary", "offset binary", "2's complement"] ("data format (offset binary)")
                                n1669 = Initialize Array(sgl 1.0, w4325) -> (w4322:sgl[])
                                n1670 = Reciprocal(x=w4331) -> (1/x=w4332:sgl)
                                n1671 = Bundle By Name("Y"=w4322, "dt"=w4332) -> (w4327:waveform(sgl))  [unwired: 1 in]
                                n1672 = call-poly <vilib>:"Analog to Digital.vi"("data format (offset binary)"=w4329, "compress digital (T)"=TRUE, "full-scale range (pk-pk)"=1.0, "resolution (16 bit)"=1, "analog waveform"=w4327) -> ("digital waveform"=w4326:digitalwaveform)  [unwired: 3 in, 3 out]
                                }
                                frame True {
                                w4339 = u16 0 items=["unsigned binary", "offset binary", "2's complement"] ("data format (offset binary)")
                                n1673 = To Double Precision Float(number=w4340) -> (double precision float=w4345:dbl)
                                n1674 = Initialize Array(sgl 1.0, w4340) -> (w4333:sgl[])
                                n1675 = Divide(x=w4344, y=w4345) -> (x/y=w4342:dbl)
                                n1676 = Round Toward +Infinity(x=w4342) -> (ceil(x): smallest int >= x=w4343:dbl)
                                n1677 = for {
                                N: w4343 -> [_]
                                tunnel: w4333 -> [w4349]
                                tunnel: [w4349] -> w4346 mode=concatenating
                                }
                                n1678 = Reciprocal(x=w4347) -> (1/x=w4348:sgl)
                                n1679 = Bundle By Name("Y"=w4346, "dt"=w4348) -> (w4337:waveform(sgl))  [unwired: 1 in]
                                n1680 = call-poly <vilib>:"Analog to Digital.vi"("data format (offset binary)"=w4339, "compress digital (T)"=TRUE, "full-scale range (pk-pk)"=1.0, "resolution (16 bit)"=1, "analog waveform"=w4337) -> ("digital waveform"=w4336:digitalwaveform)  [unwired: 3 in, 3 out]
                                }
                                }
                                n1681 = Build Array (concatenate)(w4313, w4315) -> (w4311:digitalwaveform[])
                                n1682 = call "waveformsDObuffer.vi"("DO wf in"=w4311, "command"="set") -> ()  [unwired: 1 out]
                                }
                                frame 2 {
                                n1683 = call "waveformsDObuffer.vi"("command"="get") -> ("DO wf out"=w4354:digitalwaveform[])  [unwired: 1 in]
                                n1684 = Delete From Array(array=w4354, length=1, index=w4352) -> (deleted portion=w4351:digitalwaveform[], array with subset deleted=w4350:digitalwaveform[])
                                n1685 = call "waveformsDObuffer.vi"("DO wf in"=w4350, "command"="set") -> ()  [unwired: 1 out]
                                }
                                frame 3, Default {
                                }
                                frame 0 {
                                n1686 = call "2pparameters.vi"("command"="get") -> ("params out"=w4361:T11)  [unwired: 1 in]
                                n1687 = Unbundle By Name(w4361) -> ("autoshutter"=w4360:bool, "wavdet"=w4358:bool)
                                n1688 = case shown="True" w4360 {
                                tunnel: w4359 -> [_ w4365]
                                tunnel: w4358 -> [_ w4364]
                                tunnel: [_ w4363] -> w4357
                                frame False {
                                }
                                frame True {
                                n1689 = case shown="False" w4364 {
                                tunnel: w4365 -> [w4369 _]
                                tunnel: [w4367 _] -> w4363
                                frame False {
                                w4376 = u16 0 items=["unsigned binary", "offset binary", "2's complement"] ("data format (offset binary)")
                                n1690 = call "2pparameters.vi"("command"="get") -> ("params out"=w4383:T11)  [unwired: 1 in]
                                n1691 = call "waveformsDObuffer.vi"("command"="get") -> ("DO wf out"=w4370:digitalwaveform[])  [unwired: 1 in]
                                n1692 = Unbundle By Name(w4383) -> ("Pel"=w4385:sgl, "srate"=w4384:sgl)
                                n1693 = Index Array(array=w4370, index=w4369) -> (element=w4368:digitalwaveform)
                                n1694 = Build Array(w4368) -> (w4367:digitalwaveform[])
                                n1695 = Initialize Array(sgl 1.0, w4385) -> (w4371:sgl[])
                                n1696 = Reciprocal(x=w4384) -> (1/x=w4378:sgl)
                                n1697 = Bundle By Name("Y"=w4371, "dt"=w4378) -> (w4374:waveform(sgl))  [unwired: 1 in]
                                n1698 = call-poly <vilib>:"Analog to Digital.vi"("data format (offset binary)"=w4376, "compress digital (T)"=TRUE, "full-scale range (pk-pk)"=1.0, "resolution (16 bit)"=1, "analog waveform"=w4374) -> ("digital waveform"=w4381:digitalwaveform)  [unwired: 3 in, 3 out]
                                n1699 = Replace Array Subset(array=w4370, new element=w4381, index=w4369) -> (w4366:digitalwaveform[])
                                n1700 = call "waveformsDObuffer.vi"("DO wf in"=w4366, "command"="set") -> ()  [unwired: 1 out]
                                }
                                frame True {
                                }
                                }
                                }
                                }
                                }
                                }
                                }
                                frame #8 {
                                n1701 = Build Array(w4389, w4388) -> (w4391:bool[])
                                n1702 = Boolean Array To Number(Boolean array=w4391) -> (number=w4390:u32)
                                n1703 = case shown="0" w4390 {
                                tunnel: w4387 -> [_ w4417 _ w4429]
                                tunnel: [_ w4416 _ w4427] -> w4386
                                frame 1 {
                                w4404 = 0.0 ("DOtab")
                                n1704 = call "2pparameters.vi"("command"="get") -> ("params out"=w4402:T11)  [unwired: 1 in]
                                n1705 = call "waveformparamsv2.vi"("command"="get") -> ("Params out"=w4412:T15)  [unwired: 4 in, 2 out]
                                n1706 = Unbundle By Name(w4412) -> ("DO parameters"=w4410:T18)
                                n1707 = Unbundle By Name(w4402) -> ("srate"=w4399:sgl, "Pel"=w4401:sgl)
                                n1708 = To Double Precision Float(number=w4399) -> (double precision float=w4397:dbl)
                                n1709 = To Double Precision Float(number=w4399) -> (double precision float=w4398:dbl)
                                n1710 = To Double Precision Float(number=w4401) -> (double precision float=w4393:dbl)
                                n1711 = Divide(x=w4398, y=w4393) -> (x/y=w4400:dbl)
                                n1712 = Index Array(array=w4410, index=0) -> (element=w4409:T19)
                                n1713 = Divide(x=1.0 ("Digital DC (%)"), y=w4393) -> (x/y=w4395:dbl)
                                n1714 = Multiply(x=100.0, y=w4395) -> (x*y=w4392:dbl)
                                n1715 = Bundle By Name(cluster=w4409, "Digital DC (%)"=w4392, "Digital phase"=w4404, "Digital Freq (Hz)"=w4400, "Sampling frequency (Hz)"=w4397, "Digital time offset (s)"=w4404, "padding value"=0.0, "matlab wave file"=path "LT", "DOtab"=0.0) -> (w4407:T19)
                                n1716 = Build Array(w4407) -> (w4406:T18)
                                n1717 = call "waveformparamsv2.vi"("command"="add DO", "add DO"=w4406) -> ()  [unwired: 3 in, 3 out]
                                }
                                frame 2 {
                                n1718 = call "waveformparamsv2.vi"("command"="get") -> ("Params out"=w4419:T15)  [unwired: 4 in, 2 out]
                                n1719 = in-place {
                                in-place-border: w4417 -> [w4423]
                                in-place-border: [w4422] -> w4416
                                n1720 = in-place-cluster #30(w4419) -> ("DO parameters"=w4425:T18)
                                n1721 = Delete From Array(array=w4425, length=1, index=w4423) -> (deleted portion=w4422:T18, array with subset deleted=w4424:T18)
                                n1722 = in-place-cluster #30("DO parameters"=w4424) -> (w4418:T15)
                                }
                                n1723 = call "waveformparamsv2.vi"("command"="set", "Params in"=w4418) -> ()  [unwired: 3 in, 3 out]
                                }
                                frame 3, Default {
                                }
                                frame 0 {
                                n1724 = local read "Measurement"() -> (w4431:T4)
                                n1725 = To Unsigned Long Integer(number=w4431) -> (unsigned 32bit integer=w4430:u32)
                                n1726 = case shown="5..7" w4430 {
                                tunnel: w4429 -> [_ w4433]
                                tunnel: [_ w4432] -> w4428
                                frame 0..4, Default {
                                }
                                frame 5..7 {
                                n1727 = stacked-sequence {
                                tunnel: w4433 -> [w4435 w4444]
